vi "转字符串.vi"(1 "输入":dbl) -> (0 "结果字符串":string)   [LabVIEW 2016]
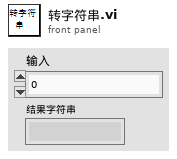
[diagram p1: front panel]
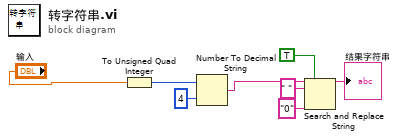
[diagram p0: block diagram]
diagram:
  n1 = To Unsigned Quad Integer(1:"输入") -> (0:w7:u64)
  n2 = Number To Decimal String(number=w7, width (-)=i16 4 ("宽度(-)")) -> (decimal integer string=w5:string)
  n3 = Search and Replace String(replace all?=TRUE ("替换全部？(F)"), input string=w5, search string=" " ("搜索字符串"), replace string="0" ("替换字符串(\"\")")) -> (result string=→"结果字符串":string)  [unwired: 4 in, 3 out]
